vi "SwaySensorMeasurments.vi"() -> ()   [LabVIEW 2014]
panel:
  out "Voltage Graph":dbl[](graph)
  out "Power Chart":dbl(graph)
  out "Current Chart":dbl(graph)
  out "Voltage Chart":dbl(graph)
  out "Power":dbl
  out "Current":dbl
  out "Voltage":dbl
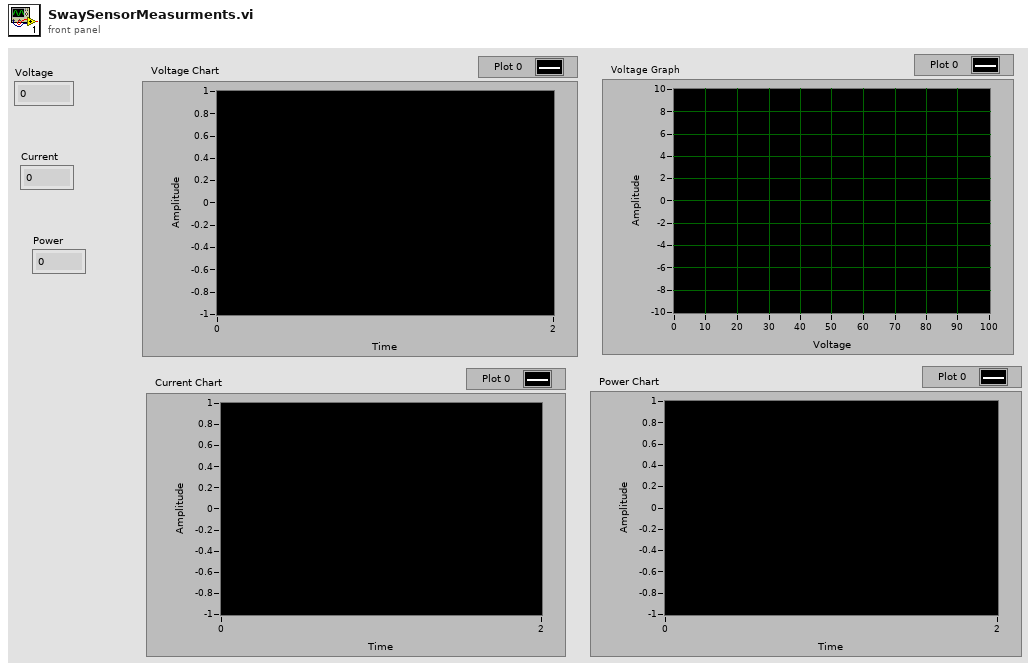
[diagram p1: front panel]
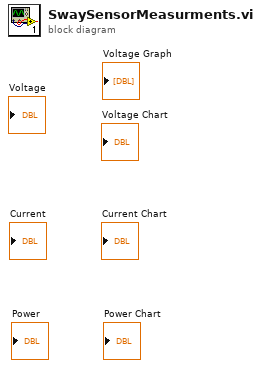
[diagram p0: block diagram]
diagram:
